vi "BuildPacket.vi"(2 "Volt 6":u16, 3 "Volt 5":u16, 4 "Actuatot GTS":i8 min=0 max=1, 5 "Sensor GTS":u8, 6 "Volt 4":u16, 7 "Volt2":u16, 8 "Volt 3":u16, 9 "Volt1":u16) -> (0 "PacketArray":i32[](array[numeric]), 1 "Packet for printing":i32[](array[numeric]))   [LabVIEW 2011]
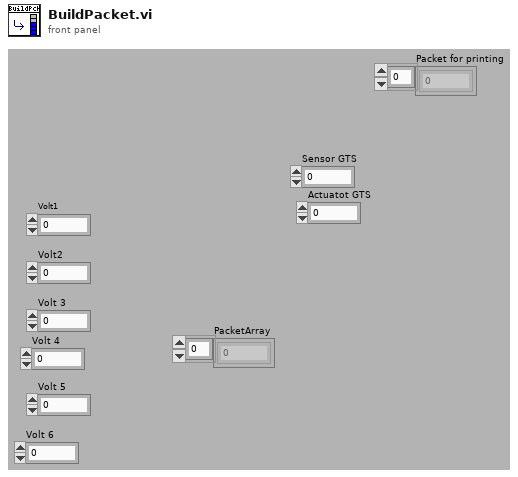
[diagram p1: front panel]
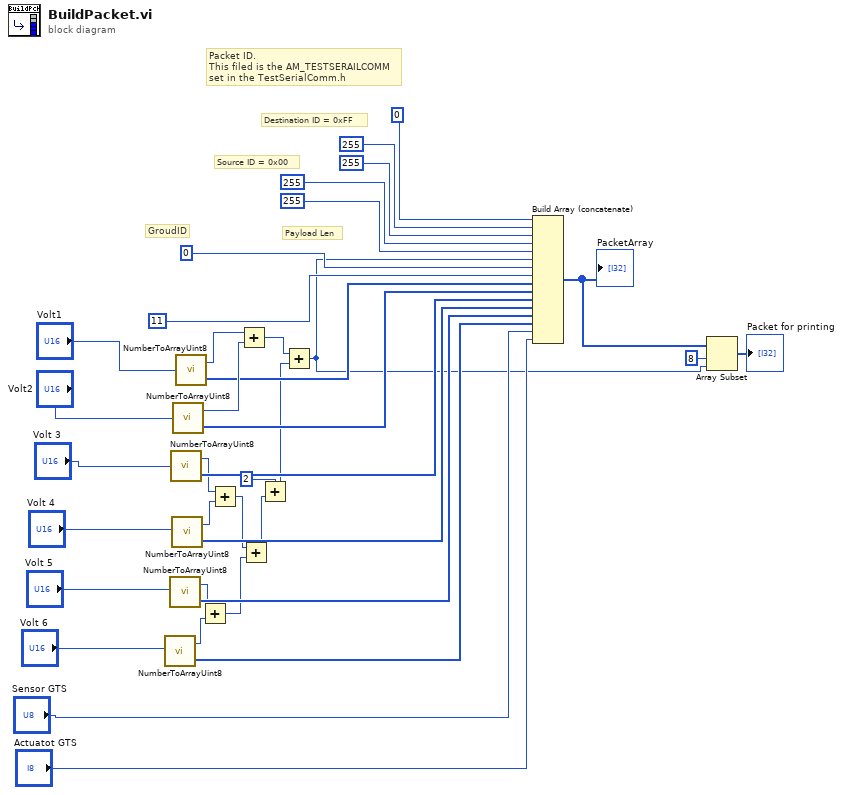
[diagram p0: block diagram]
diagram:
  # "Packet ID.\nThis filed is the AM_TESTSERAILCOMM \nset in the TestSerialComm.h"
  # "GroudID"
  # "Payload Len"
  # "Source ID = 0x00"
  # "Destination ID = 0xFF"
  n1 = call "NumberToArrayUint8.vi"("Numeric 2"="Volt 6") -> ("Array"=w14:i8[], "Numeric"=w12:i32)
  n2 = call "NumberToArrayUint8.vi"("Numeric 2"="Volt 5") -> ("Array"=w15:i8[], "Numeric"=w13:i32)
  n3 = call "NumberToArrayUint8.vi"("Numeric 2"="Volt 3") -> ("Array"=w20:i8[], "Numeric"=w11:i32)
  n4 = call "NumberToArrayUint8.vi"("Numeric 2"="Volt 4") -> ("Array"=w16:i8[], "Numeric"=w10:i32)
  n5 = call "NumberToArrayUint8.vi"("Numeric 2"="Volt2") -> ("Array"=w33:i8[], "Numeric"=w35:i32)
  n6 = call "NumberToArrayUint8.vi"("Numeric 2"="Volt1") -> ("Array"=w32:i8[], "Numeric"=w34:i32)
  n7 = Add(x=w13, y=w12) -> (x+y=w8:i32)
  n8 = Add(x=w11, y=w10) -> (x+y=w9:i32)
  n9 = Add(x=w34, y=w35) -> (x+y=w24:i32)
  n10 = Add(x=w9, y=w8) -> (x+y=w7:i32)
  n11 = Add(x=2, y=w7) -> (x+y=w5:i32)
  n12 = Add(x=w24, y=w5) -> (x+y=w2:i32)
  n13 = Build Array (concatenate)(0, 255, 255, 255, 255, w2, 0, i8 11, w32, w33, w20, w16, w15, w14, "Sensor GTS", "Actuatot GTS") -> (w4:i32[])
  "PacketArray" <- w4
  n14 = Array Subset(array=w4, index=8, length=w2) -> (→"Packet for printing":i32[])
